vi "Launch.vi"(4 "Sub Panel":refnum<vi>, 6 "Name":string="Metronome", 7 "Front Panel State (Hidden)":T1=enum."Hidden", 8 "error in (no error)":errorcluster, 10 "Period [ms]":i32, 11 "Response Channel":refnum<class "Messenger.lvclass">) -> (0 "error out":errorcluster, 3 "Actor API":refnum<class "Metronome Actor API.lvclass">)   [LabVIEW 2015, in "Metronome Actor.lvclass"]
doc: "<b>Response</b> channel is used by this actor to return infomation back to the parent. Typically this input is the Request channel of the parent actor."
uses:
  Metronome Actor.lvclass
  Messaging/Messenger/Messenger.lvclass
  Base Actor/Actor/Front Panel State.ctl
  API/Metronome Actor API.lvclass
  Metronome Actor.lvclass/Metronome Actor.ctl
  Base Actor/Actor/Actor.lvclass
  Base Actor/API/Actor API.lvclass
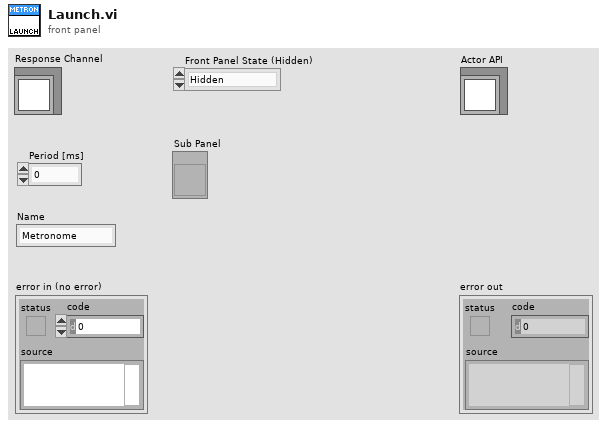
[diagram p1: front panel]
types:
  T1 = typedef "Actor.lvclass/Front Panel State.ctl" = enum32{"Invalid", "Standard", "Closed", "Hidden", "Minimized", "Maximized"}
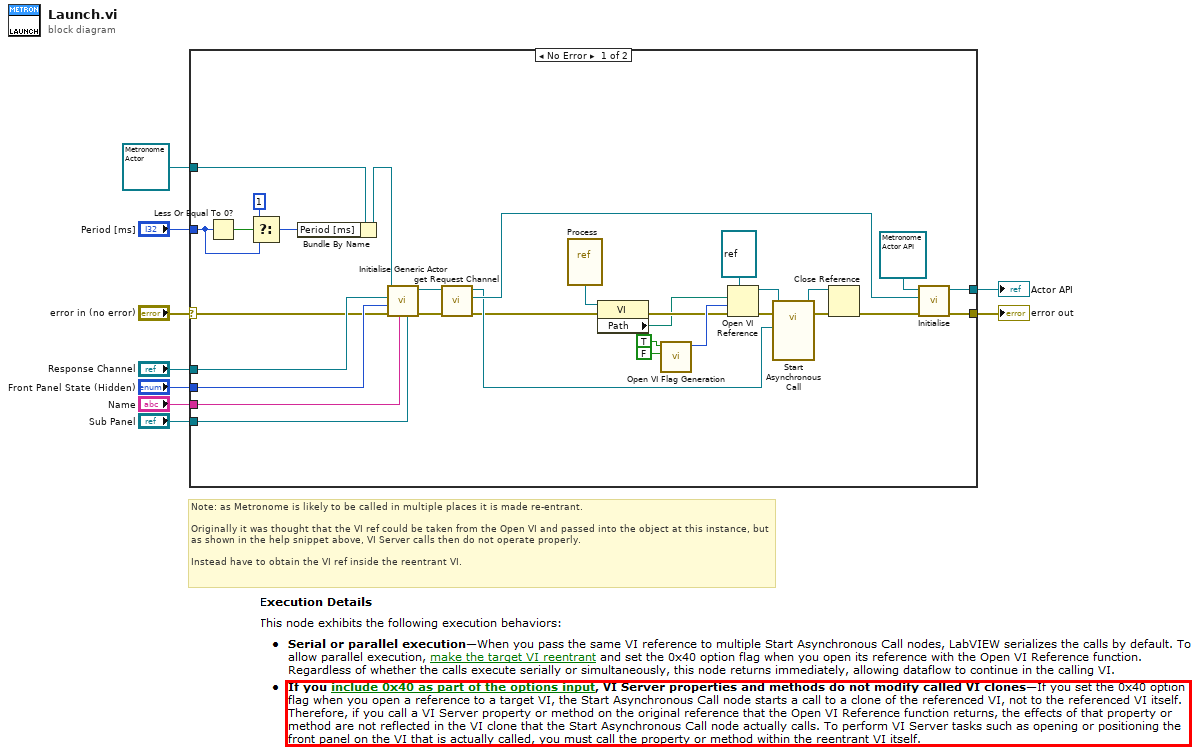
[diagram p0: block diagram]
diagram:
  # "Note: as Metronome is likely to be called in multiple places it is made re-entrant. \n\nOriginally it was thought that the VI ref could be taken from the Open VI and passed into the object at this instance, but as shown in the help snippet above, VI Server calls then do not operate properly.\n\nInstead have to obtain the VI ref inside the reentrant VI."
  n1 = case shown="No Error" "error in (no error)" {
    selector: "error in (no error)" -> [w23 w40]
    tunnel: [w19 w40] -> w9
    tunnel: "Response Channel" -> [w35 _]
    tunnel: refnum<class "Metronome Actor.lvclass"> refnum ("Worker Test 1.lvclass") -> [w34 _]
    tunnel: "Period [ms]" -> [w15 _]
    tunnel: "Name" -> [w32 _]
    tunnel: "Front Panel State (Hidden)" -> [w31 _]
    tunnel: [w26 _] -> w2
    tunnel: "Sub Panel" -> [w18 _]
    frame No Error {
      n2 = Less Or Equal To 0?(x=w15) -> (x <= 0?=w17:bool)
      n3 = Select(t=1 ("Period [ms]"), s=w17, f=w15) -> (s? t:f=w14:i32)
      n4 = Bundle By Name(cluster=w34, "Period [ms]"=w14) -> (w33:refnum<class "Metronome Actor.lvclass">)
      n5 = call-dynamic "Initialise Generic Actor.vi"("Sub Panel"=w18, "Name"=w32, "Front Panel State"=w31, "Response Channel"=w35, "Actor in"=w33) -> ("Actor out"=w22:refnum<class "Metronome Actor.lvclass">)  [unwired: 5 in, 1 out]
      n6 = call "get Request Channel.vi"("error in (no error)"=w23, "Actor in"=w22) -> ("error out"=w13:errorcluster, "Request Channel"=w24:refnum<class "Messenger.lvclass">, "Actor out"=w21:refnum<class "Metronome Actor.lvclass">)  [unwired: 7 in]
      n7 = vi-ref "Process.vi"() -> (w11:refnum<vi>)
      n8 = property class="VI"(reference=w11, error in=w13) -> (error out=w12:errorcluster, "Path"=w10:path)  [unwired: 1 out]
      n9 = call "Open VI Flag Generation.vi"("Call And Collect (F)"=FALSE, "Re-entrant (F)"=TRUE) -> ("Flags"=w39:i32)  [unwired: 9 in]
      n10 = Open VI Reference(type specifier VI Refnum (for type only)=refnum<vi> refnum, vi path=w10, options=w39, error in (no error)=w12) -> (vi reference=w30:refnum<vi>, error out=w29:errorcluster)  [unwired: 2 in]
      n11 = call-by-ref "Start Asynchronous Call"(reference=w30, error in=w29, "Worker Test 1.lvclass"=w21) -> (reference out=w27:refnum<vi>, error out=w28:errorcluster)  [unwired: 11 in]
      n12 = Close Reference(reference=w27, error in (no error)=w28) -> (error out=w20:errorcluster)
      n13 = call "Initialise.vi"("error in (no error)"=w20, "Request Channel"=w24, "Actor API in"=refnum<class "Metronome Actor API.lvclass"> refnum ("Actor API")) -> ("error out"=w19:errorcluster, "Actor API out"=w26:refnum<class "Metronome Actor API.lvclass">)  [unwired: 7 in]
    }
    frame Error {
    }
  }
  "error out" <- w9
  "Actor API" <- w2
